vi "IsUserAnAdmin.vi"(8 "error in (no error)":errorcluster) -> (0 "error out":errorcluster, 2 "Administrator":bool)   [LabVIEW 2017]
doc: "Returns TRUE when the current process is running with administrator rights."
uses:
  shell32.dll
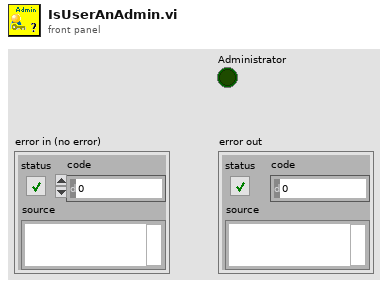
[diagram p1: front panel]
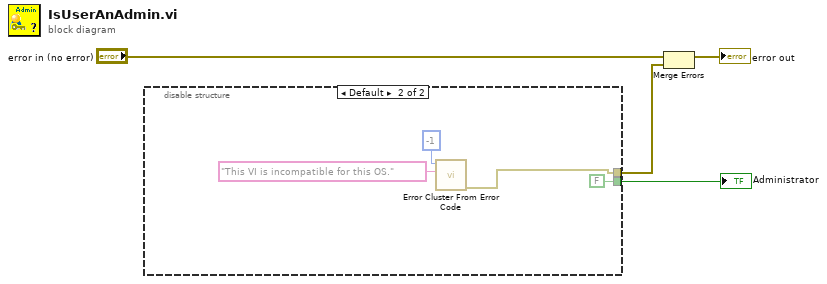
[diagram p0: block diagram]
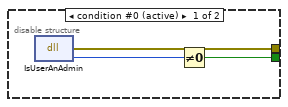
[diagram p2: hidden frame]
diagram:
  n1 = disable-structure shown="Default" {
    disable-tunnel: [w7 w8] -> w2
    disable-tunnel: [w5 FALSE] -> w1
    frame condition #0 (active) {
      n2 = dll-call lib="shell32.dll" fn="IsUserAnAdmin"() -> (error out=w7:errorcluster, "return type"=w6:i32)  [unwired: 3 in, 1 out]
      n3 = Not Equal To 0?(x=w6) -> (x != 0?=w5:bool)
    }
    frame condition #1 {
      n4 = call <vilib>:"Error Cluster From Error Code.vi"("error message (\"\")"="This VI is incompatible for this OS." ("error message (\"\")"), "error code (0)"=-1) -> ("error out"=w8:errorcluster)  [unwired: 7 in]
    }
  }
  "Administrator" <- w1
  n5 = Merge Errors("error in (no error)", w2) -> (→"error out":errorcluster)
